vi "1-Hindbrain.vi"() -> ()   [LabVIEW 2010]
doc: "Hindbrain_RobotBrainExample. This VI is an example of the Hindbrain layer of the Olin Robot Architecture. It collects all SENSE data and sends it up three neural clusters to the Midbrain and accepts one ACT cluster from Midbrain to drive all robot actuators. \n\nTo start the program press the run arrow and then press \"Begin\""
uses:
  2-Low Neurons/2.2-Where Sensor Typedef.ctl
  2-Low Neurons/2.3-What Sensor Typedef.ctl
  2-Low Neurons/Data Latch.ctl
  2-Low Neurons/2.4-How Sensor Typedef.ctl
  2-Low Neurons/2.1-Act Command Typedef.ctl
  2-Low Neurons/2.0-Hindbrain Startup State.ctl
  <vilib>/eio/EIONode/EIONode.xnode
  <vilib>/rvi/eio/nirviEIOImplementation/nirviEIOImplementation.xnode
  <vilib>/rvi/eio/common/nirviEmuClasses.ctl
  1-Hindbrain/1.0-Hindbrain Global.vi
  <vilib>/rvi/eio/common/nirviEmuTemplateMethod_noerrors.vi
panel:
  in  "Blinking light blink rate":u32(slide) scale=100.0..500.0
  in  "Restart":bool
  out "1.0-Hindbrain State":T1
  in  "Begin":bool
  in  "2.1 Act Command":T2
  out "2.4 How Am I? Sensor":T3
  out "2.3 What is Around Me? Sensor":T4={"FPGA Raw Datalatch"=enum."Idle", "Drivable Path Integers"=[0, 0, 0, 0, 0, 0, 0, 0, 0, 0, 0, 0, 0, 0, 0, 0]}
  out "2.2 Where am I? Sensor":T6
  out "HeartBeat":bool
  in  "stop":bool
  # "To start the  program press  the run arrow and then press \"Begin\""
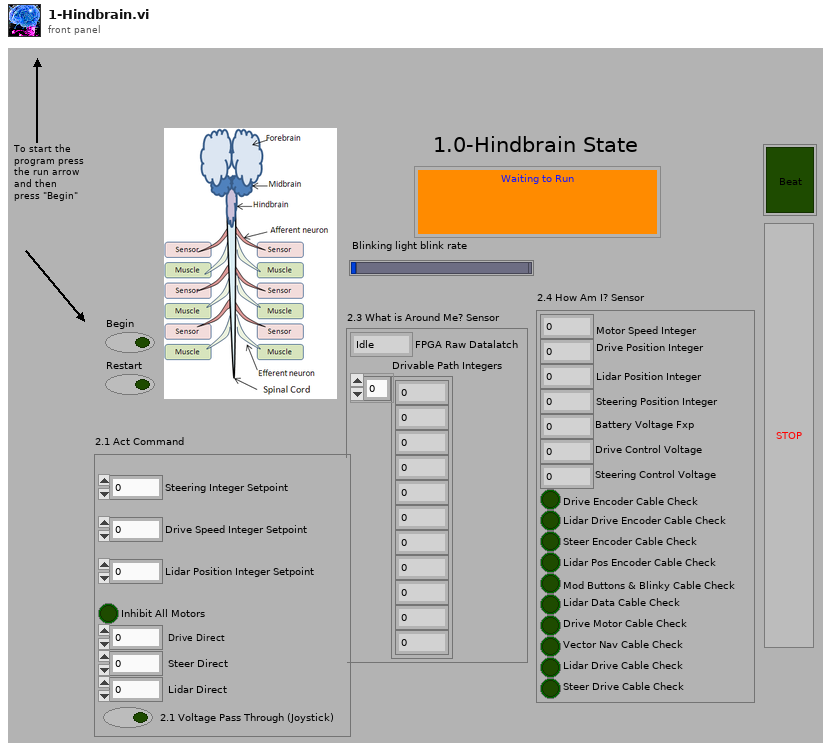
[diagram p1: front panel]
types:
  T1 = typedef "2.0-Hindbrain Startup State.ctl" = enum8{"Waiting to Run", "Running", "Restart", "Shutdown", "Off"}
  T2 = typedef "2.1-Act Command Typedef.ctl" = cluster{"Steering Integer Setpoint":i16, "Drive Speed Integer Setpoint":i16, "Lidar Position Integer Setpoint":i16, "Inhibit All Motors":bool, "Drive Direct":fxp<+/-,20,5>, "Steer Direct":fxp<+/-,20,5>, "Lidar Direct ":fxp<+/-,20,5>, "2.1 Voltage Pass Through (Joystick)":bool}
  T3 = typedef "2.4-How Sensor Typedef.ctl" = cluster{"Motor Speed Integer":i16, "Drive Position Integer":i32, "Lidar Position Integer":i32, "Steering Position Integer":i32, "Battery Voltage Fxp":fxp<+/-,16,5>, "Drive Control Voltage":fxp<+/-,20,5>, "Steering Control Voltage":fxp<+/-,20,5>, "Drive Encoder Cable Check":bool, "Lidar Drive Encoder Cable Check":bool, "Steer Encoder Cable Check":bool, "Lidar Pos Encoder Cable Check":bool, "Mod Buttons & Blinky Cable Check":bool, "Lidar Data Cable Check":bool, "Drive Motor Cable Check":bool, "Vector Nav Cable Check":bool, "Lidar Drive Cable Check":bool, "Steer Drive Cable Check":bool}
  T4 = typedef "2.3-What Sensor Typedef.ctl" = cluster{"FPGA Raw Datalatch":T5, "Drivable Path Integers":u16[]}
  T5 = typedef "Data Latch.ctl" = enum8{"Idle", "Sending", "Sent", "Receiving", "Received"}
  T6 = typedef "2.2-Where Sensor Typedef.ctl" = cluster{"INS X":i16, "INS Y":i16, "INS Z":i16, "INS Yaw":i16}
  T7 = typedef "nirviEmuClasses.ctl" = enum16{"IO Read", "IO Write", "Method", "Property Read", "Property Write"}
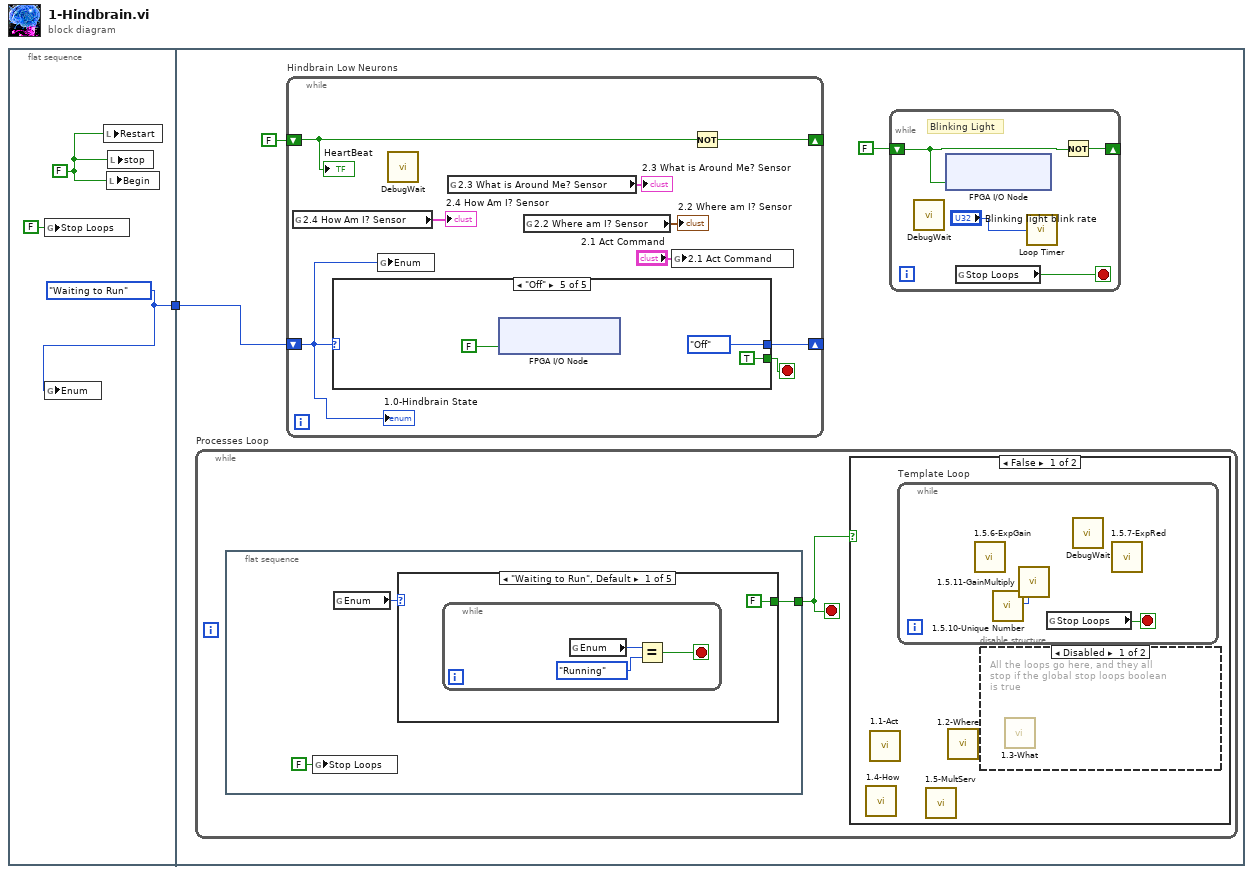
[diagram p0: block diagram]
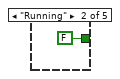
[diagram p4: hidden frame]
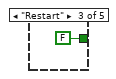
[diagram p5: hidden frame]
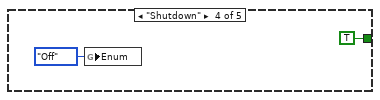
[diagram p6: hidden frame]
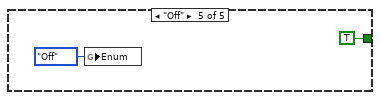
[diagram p7: hidden frame]
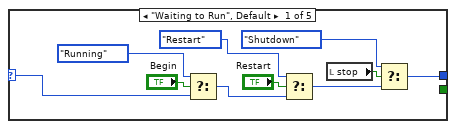
[diagram p8: hidden frame]
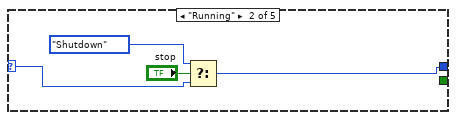
[diagram p9: hidden frame]
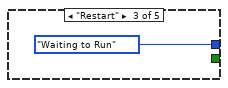
[diagram p10: hidden frame]
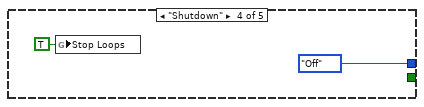
[diagram p11: hidden frame]
diagram:
  n1 = flat-sequence {
    tunnel: [w3] -> w1
    tunnel: w1 -> [w7]
    frame #0 {
      w3 = 2.0-Hindbrain_Startup_State."Waiting to Run" ("Enum")
      w2 = FALSE
      n2 = global write "1.0-Hindbrain Global.vi" "Stop Loops"(FALSE ("Stop Loops")) -> ()
      n3 = global write "1.0-Hindbrain Global.vi" "Enum"(w3) -> ()
      n4 = local write "Restart"(w2) -> ()
      n5 = local write "Begin"(w2) -> ()
      n6 = local write "stop"(w2) -> ()
    }
    frame #1 {
      n7 = while "Processes Loop" {
        stop <- w23 stop-if-true
        n8 = flat-sequence {
          tunnel: [w27] -> w23
          frame #0 {
            n9 = global write "1.0-Hindbrain Global.vi" "Stop Loops"(FALSE ("Stop Loops")) -> ()
            n10 = global read "1.0-Hindbrain Global.vi" "Enum"() -> (w28:T1)
            n11 = case shown="\"Waiting to Run\", Default" w28 {
              tunnel: [FALSE FALSE FALSE TRUE TRUE] -> w27
              frame "Waiting to Run", Default {
                n12 = while {
                  stop <- w30 stop-if-true
                  n13 = global read "1.0-Hindbrain Global.vi" "Enum"() -> (w32:T1)
                  n14 = Equal?(x=w32, y=2.0-Hindbrain_Startup_State."Running") -> (x = y?=w30:bool)
                }
              }
              frame "Running" {
              }
              frame "Restart" {
              }
              frame "Shutdown" {
                n15 = global write "1.0-Hindbrain Global.vi" "Enum"(2.0-Hindbrain_Startup_State."Off" ("Enum")) -> ()
              }
              frame "Off" {
                n16 = global write "1.0-Hindbrain Global.vi" "Enum"(2.0-Hindbrain_Startup_State."Off" ("Enum")) -> ()
              }
            }
          }
        }
        n17 = case shown="False" w23 {
          frame False {
            n18 = call "1.4-How.vi"() -> ()  [unwired: 12 in]
            n19 = call "1.1-Act.vi"() -> ()  [unwired: 12 in]
            n20 = while "Template Loop" {
              stop <- w25 stop-if-true
              n21 = call "1.5.6-ExpGain.vi"() -> ()  [unwired: 2 in, 1 out]
              n22 = call "1.5.10-Unique Number.vi"() -> ("Number"=w24:u8)
              n23 = call "1.5.11-GainMultiply.vi"("Unique 8b identifier"=w24) -> ()  [unwired: 12 in, 3 out]
              n24 = global read "1.0-Hindbrain Global.vi" "Stop Loops"() -> (w25:bool)
              n25 = call "DebugWait.vi"() -> ()  [unwired: 12 in]
              n26 = call "1.5.7-ExpRed.vi"() -> ()  [unwired: 2 in, 1 out]
            }
            n27 = call "1.5-MultServ.vi"() -> ()  [unwired: 12 in]
            n28 = call "1.2-Where.vi"() -> ()  [unwired: 12 in]
            n29 = disable-structure shown="Disabled" {
              frame Disabled {
                # "All the loops go here, and they all\nstop if the global stop loops boolean\nis true"
                n30 = call "1.3-What.vi"() -> ()  [unwired: 12 in]
              }
              frame Enabled {
              }
            }
          }
          frame True {
          }
        }
      }
      n31 = while "Hindbrain Low Neurons" {
        shift-right: [w43] -> _
        shift-left: w7 -> [w41]
        shift-right: [w39] -> _
        shift-left: FALSE -> [w40]
        stop <- w42 stop-if-true
        n32 = global read "1.0-Hindbrain Global.vi" "2.4 How Am I? Sensor"() -> (→"2.4 How Am I? Sensor":T3)
        n33 = case shown="\"Off\"" w41 {
          selector: w41 -> [w54 w60 _ _ _]
          tunnel: [w56 w59 2.0-Hindbrain_Startup_State."Waiting to Run" ("Enum") 2.0-Hindbrain_Startup_State."Off" ("Enum") 2.0-Hindbrain_Startup_State."Off" ("Enum")] -> w43
          tunnel: [_ _ _ _ TRUE] -> w42
          frame "Waiting to Run", Default {
            n34 = Select(t=2.0-Hindbrain_Startup_State."Running", s="Begin", f=w54) -> (s? t:f=w51:T1)
            n35 = Select(t=2.0-Hindbrain_Startup_State."Restart", s="Restart", f=w51) -> (s? t:f=w50:T1)
            n36 = local read "stop"() -> (w55:bool)
            n37 = Select(t=2.0-Hindbrain_Startup_State."Shutdown", s=w55, f=w50) -> (s? t:f=w56:T1)
          }
          frame "Running" {
            n38 = Select(t=2.0-Hindbrain_Startup_State."Shutdown", s="stop", f=w60) -> (s? t:f=w59:T1)
          }
          frame "Restart" {
          }
          frame "Shutdown" {
            n39 = global write "1.0-Hindbrain Global.vi" "Stop Loops"(TRUE ("Stop Loops")) -> ()
          }
          frame "Off" {
            n40 = xnode "FPGA I/O Node"("Not E-Stopped"=FALSE) -> ()  [unwired: 1 in, 1 out]
          }
        }
        n41 = global write "1.0-Hindbrain Global.vi" "Enum"(w41) -> ()
        n42 = call "DebugWait.vi"() -> ()  [unwired: 12 in]
        n43 = global read "1.0-Hindbrain Global.vi" "2.3 What is Around Me? Sensor"() -> (→"2.3 What is Around Me? Sensor":T4)
        n44 = global read "1.0-Hindbrain Global.vi" "2.2 Where am I? Sensor"() -> (→"2.2 Where am I? Sensor":T6)
        n45 = global write "1.0-Hindbrain Global.vi" "2.1 Act Command"("2.1 Act Command") -> ()
        n46 = Not(x=w40) -> (.not. x?=w39:bool)
        "HeartBeat" <- w40
        "1.0-Hindbrain State" <- w41
      }
      n47 = while {
        shift-right: [w11] -> _
        shift-left: FALSE -> [w10]
        stop <- w9 stop-if-true
        # "Blinking Light"
        n48 = call "DebugWait.vi"() -> ()  [unwired: 12 in]
        n49 = xnode "FPGA I/O Node"("Blinky Light"=w10) -> ()  [unwired: 1 in, 1 out]
        n50 = global read "1.0-Hindbrain Global.vi" "Stop Loops"() -> (w9:bool)
        n51 = call "Loop Timer"("Count(mSec)"="Blinking light blink rate") -> ()  [unwired: 1 out]
        n52 = Not(x=w10) -> (.not. x?=w11:bool)
      }
    }
  }
